vi "Transform_Calc_A_matrix.vi"(11 "PairedFiducialCoordinates":T2[](array[typedef])) -> (0 "pinv(X')":T1, 1 "A":T1, 2 "error":i32, 4 "X'":T1, 6 "Y'":T1)   [LabVIEW 2011]
doc: "Find the matrix A that transforms shifted Reference Session Fiducials to the shifted Current Session Fiducials. This establishes the scaling and rototation transform that will transform a point from reference session to the current session. The Paired Coordinates input into this function have been shifted to have a common point of rotation. That point could be any common point in the two coordinate systems but in this case the software has shifted the first pair of fiducials in the list to the origin and the scaling and rotation is done about that point.\n\nSince theirthere may be more than 3 fiducials a psuedopseudo inverse may be applied. Labview's native PINV funcitonfunction is used to invert the matrix. The details of the transform are givegiven as: \n\nfirstFirst translate the two constalationsconstellations of fiducials so there is a common point at the origin (done in the calling routine). Stack up the translated reference and current session fiducial into a matrix where rows are the vectors (R is the rectangular matrix of translated reference fiducials and Y is the matrix of the current session fiducials). Now, since A * R = Y, the inverse or psuedopseudo inverse of R is found and multiplied on both right on both sides of the equationhand sides of the equpation to find A = Y * inv(R)."
uses:
  Fiducial_pair.ctl
  <vilib>/Analysis/Matrix/Datatypes/RealMatrix.ctl
  <vilib>/Analysis/Matrix/Numeric/Conversions/Array To Matrix - RA2.vi
  <vilib>/Analysis/_algsub.llb/Real PseudoInverse Matrix.vi
  <vilib>/Analysis/Matrix/Numeric/Multiply/Multiply - RM,RM.vi
  <vilib>/Analysis/Matrix/NI_Matrix.lvlib
  <vilib>/Analysis/NI_AALPro.lvlib
panel:
  # "y = Ax\n\n[y1 y2 y3 ... ] = A{x1 x2 x3 ...]\n\nA = [y1 y2 y3 ...] pseudo_inverse([x1 x2 x3 ..])"
  # "Fiducial Location Pair"
  # "Current Instrument Fiducial Location"
  # "Reference Instrument Fiducial Location"
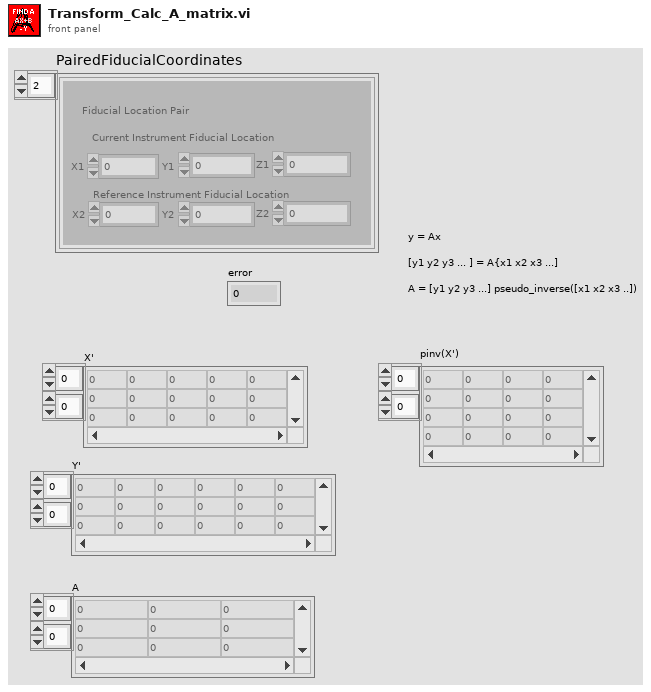
[diagram p1: front panel]
types:
  T1 = typedef "NI_Matrix.lvlib/RealMatrix.ctl" = dbl[][]
  T2 = typedef "Fiducial_pair.ctl" = cluster{"X1":dbl, "X2":dbl, "Y1":dbl, "Y2":dbl, "Z1":dbl, "Z2":dbl}
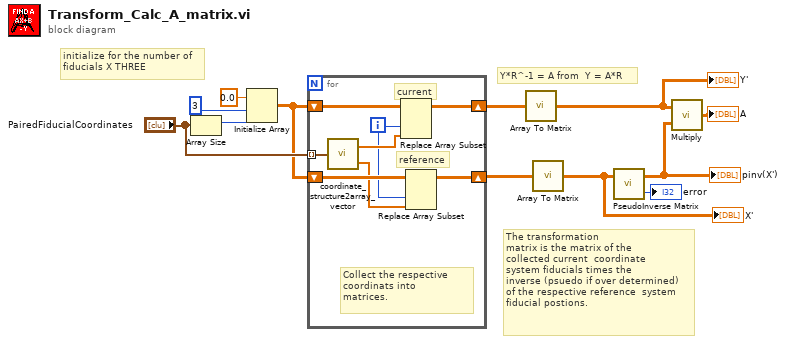
[diagram p0: block diagram]
diagram:
  # "initialize for the number of\nfiducials X THREE"
  # "Y*R^-1 = A from  Y = A*R"
  # "The transformation\nmatrix is the matrix of the\ncollected current  coordinate\nsystem fiducials times the\ninverse (psuedo if over determined)\nof the respective reference  system\nfiducial postions."
  n1 = Array Size(array="PairedFiducialCoordinates") -> (size(s)=w1:i32)
  n2 = Initialize Array(0.0 ("element"), 3 ("dimension size"), w1) -> (w6:dbl[][])
  n3 = for {
    tunnel: "PairedFiducialCoordinates" -> [w20] mode=indexing
    shift-right: [w17] -> w7
    shift-left: w6 -> [w19]
    shift-right: [w15] -> w8
    shift-left: w6 -> [w16]
    i -> [w13]
    # "reference"
    # "current"
    # "Collect the respective coordinats into\nmatrices."
    n4 = call "coordinate_structure2array_vector.vi"("Fiducial_Pos_structure"=w20) -> ("Current_Instrument_pos"=w18:dbl[], "Reference_Instrument_pos"=w14:dbl[])
    n5 = Replace Array Subset(array=w19, new element=w18, index (col)=w13) -> (w17:dbl[][])  [unwired: 1 in]
    n6 = Replace Array Subset(array=w16, new element=w14, index (col)=w13) -> (w15:dbl[][])  [unwired: 1 in]
  }
  n7 = call-poly <vilib>:"Array To Matrix.vi"("Real 2D Array"=w7) -> ("Real Matrix"=w3:T1)
  "Y'" <- w3
  n8 = call-poly <vilib>:"Array To Matrix.vi"("Real 2D Array"=w8) -> ("Real Matrix"=w4:T1)
  "X'" <- w4
  n9 = call-poly <vilib>:"PseudoInverse Matrix.vi"("Input Matrix"=w4) -> ("error"=→"error":i32, "PseudoInverse Matrix"=w10:T1)  [unwired: 1 in]
  "pinv(X')" <- w10
  n10 = call-poly <vilib>:"Multiply.vi"("Real Matrix B"=w10, "Real Matrix A"=w3) -> ("A * B"=→"A":T1)
